vi "Draw Feeder Overlay.vi"(9 "Rectangle":T1, 11 "Refnum in":T2) -> (3 "Refnum out":T2)   [LabVIEW 2015]
uses:
  <vilib>/vision/Image Controls.llb/IMAQ Image.ctl
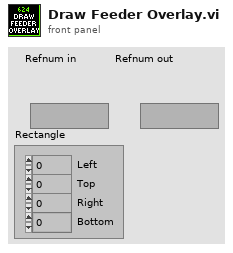
[diagram p1: front panel]
types:
  T1 = cluster{"Left":i32, "Top":i32, "Right":i32, "Bottom":i32}
  T2 = typedef "IMAQ Image.ctl" = refnum<image>
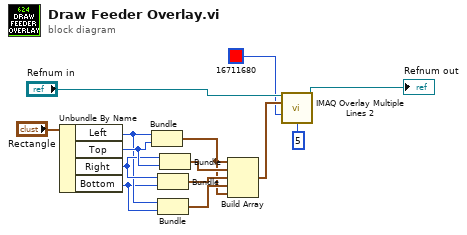
[diagram p0: block diagram]
diagram:
  n1 = Unbundle By Name("Rectangle") -> ("Left"=w9:i32, "Top"=w11:i32, "Right"=w10:i32, "Bottom"=w8:i32)
  n2 = Bundle("Left"=w9, "Top"=w11) -> (w4:cluster{"Left":i32, "Top":i32})  [unwired: 1 in]
  n3 = Bundle("Right"=w10, "Bottom"=w8) -> (w6:cluster{"Right":i32, "Bottom":i32})  [unwired: 1 in]
  n4 = Bundle("Left"=w9, "Bottom"=w8) -> (w5:cluster{"Left":i32, "Bottom":i32})  [unwired: 1 in]
  n5 = Bundle("Right"=w10, "Top"=w11) -> (w7:cluster{"Right":i32, "Top":i32})  [unwired: 1 in]
  n6 = Build Array(w4, w7, w6, w5, w4) -> (w3:cluster{"Left":i32, "Top":i32}[])
  n7 = call "IMAQ Overlay Multiple Lines 2"("Image"="Refnum in", "Line End Points"=w3, "Color"=u32 16711680, "Width"=u32 5) -> ("Image Out"=→"Refnum out":T2)  [unwired: 10 in, 1 out]
